vi "Change buffer.vi"(8 "error in (no error)":errorcluster) -> (0 "error out":errorcluster)   [LabVIEW 2018, in "cetoni.lvlib" / "cetoni.lvclass"]
uses:
  cetoni.lvclass
  Resources/GLOBAL/GLOBAL Time-critical.vi
  <userlib>/QmixLib/QmixLib.lvlib
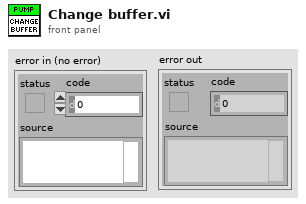
[diagram p1: front panel]
types:
  T1 = enum16{"Left Button", "Center Button", "Right Button", "Window Close"}
  T2 = enum16{"LOW_PRESSURE_VALVE", "BALL_VALVE", "QMIX_VALVE"}
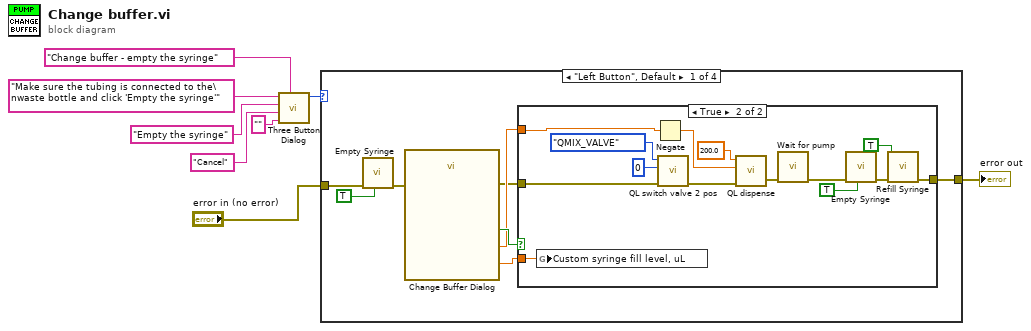
[diagram p0: block diagram]
diagram:
  n1 = call <vilib>:"Three Button Dialog.vi"("Window Title (\"\")"="Change buffer - empty the syringe" ("Window Title (\"\")"), "Right Button Text (\"Cancel\")"="" ("Right Button Text (\"Cancel\")"), "Center Button Text (\"No\")"="Cancel" ("Center Button Text (\"No\")"), "Left Button Text (\"Yes\")"="Empty the syringe" ("Left Button Text (\"Yes\")"), "message"="Make sure the tubing is connected to the\nwaste bottle and click 'Empty the syringe'") -> ("Which Button?"=w3:T1)  [unwired: 6 in]
  n2 = case shown="\"Left Button\", Default" w3 {
    tunnel: [w10 w32 w33 w34] -> w2
    tunnel: "error in (no error)" -> [w9 w32 w33 w34]
    frame "Left Button", Default {
      n3 = call "Empty Syringe.vi"("Wait for pump"=TRUE, "error in (no error)"=w9) -> ("error out"=w15:errorcluster)  [unwired: 9 in]
      n4 = call "Change Buffer Dialog.vi"("error in (no error)"=w15) -> ("Refill volume, µL"=w13:dbl, "Rinse volume, µL"=w12:dbl, "Refill"=w14:bool, "error out"=w11:errorcluster)  [unwired: 15 in]
      n5 = case shown="True" w14 {
        tunnel: w13 -> [_ w31]
        tunnel: w12 -> [_ w18]
        tunnel: w11 -> [w17 w30]
        tunnel: [w17 w21] -> w10
        frame False {
        }
        frame True {
          n6 = global write "GLOBAL Time-critical.vi" "Custom syringe fill level, uL"(w31) -> ()
          n7 = Negate(x=w18) -> (-x=w19:dbl)
          n8 = call <userlib>:"QL switch valve 2 pos.vi"("error in (no error)"=w30, "pos"=0, "valve"=T2."QMIX_VALVE") -> ("error out"=w22:errorcluster)  [unwired: 8 in]
          n9 = call <userlib>:"QL dispense.vi"("error in (no error)"=w22, "volume_uL"=w19, "flow_rate_uL_s"=200.0) -> ("error out"=w27:errorcluster)  [unwired: 4 in]
          n10 = call "Wait for pump.vi"("error in (no error)"=w27) -> ("error out"=w28:errorcluster)  [unwired: 10 in]
          n11 = call "Empty Syringe.vi"("Wait for pump"=TRUE, "error in (no error)"=w28) -> ("error out"=w25:errorcluster)  [unwired: 9 in]
          n12 = call "Refill Syringe.vi"("error in (no error)"=w25, "Wait for pump"=TRUE) -> ("error out"=w21:errorcluster)  [unwired: 9 in]
        }
      }
    }
    frame "Center Button" {
    }
    frame "Right Button" {
    }
    frame "Window Close" {
    }
  }
  "error out" <- w2
